vi "2-DIOConfig.vi"(8 "error in (no error)":errorcluster caption="错误输入（无错误）", 10 "DIO pra in":T1, 11 "Step":enum16{"Initial", "Write", "Read"}(ring)) -> (0 "error out":errorcluster caption="错误输出", 3 "DIO pra out":T1)   [LabVIEW 2017]
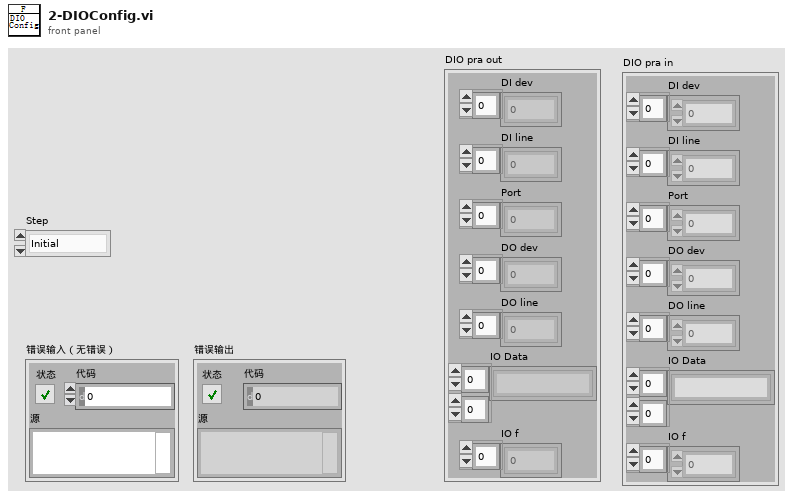
[diagram p1: front panel]
types:
  T1 = cluster{"DI dev":i32[], "DI line":i32[], "Port":i32[], "DO dev":i32[], "DO line":i32[], "IO Data":string[][], "IO f":i16[]}
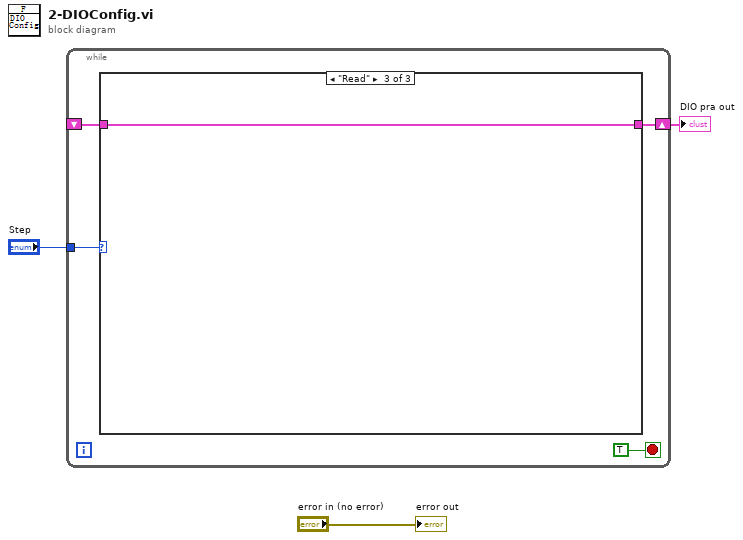
[diagram p0: block diagram]
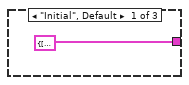
[diagram p2: hidden frame]
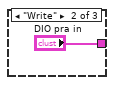
[diagram p3: hidden frame]
diagram:
  n1 = while {
    tunnel: "Step" -> [w7]
    shift-right: [w5] -> w1
    shift-left: _ -> [w4]
    stop <- TRUE stop-if-true
    n2 = case shown="\"Read\"" w7 {
      tunnel: [T1 {"DI dev"=[], "DI line"=[], "Port"=[], "DO dev"=[], "DO line"=[], "IO Data"=[], "IO f"=[]} ("IO pra in") "DIO pra in" w10] -> w5
      tunnel: w4 -> [_ _ w10]
      frame "Initial", Default {
      }
      frame "Write" {
      }
      frame "Read" {
      }
    }
  }
  "DIO pra out" <- w1
  "error out" <- "error in (no error)"
